vi "Init.vi"(0 "Session Handle in":T1, 11 "error in (no error)":errorcluster) -> (4 "Session Handle out":T1, 15 "error out":errorcluster)   [LabVIEW 2019, in "SmartScopeDriver.lvclass"]
doc: "Initializes the Smart Scope."
uses:
  SmartScopeDriver.lvclass
  Typedefs/Session Handle.ctl
  SmartScopeDriver.lvclass/SmartScopeDriver.ctl
  Scope Driver/LabNation Scope Driver.lvlib
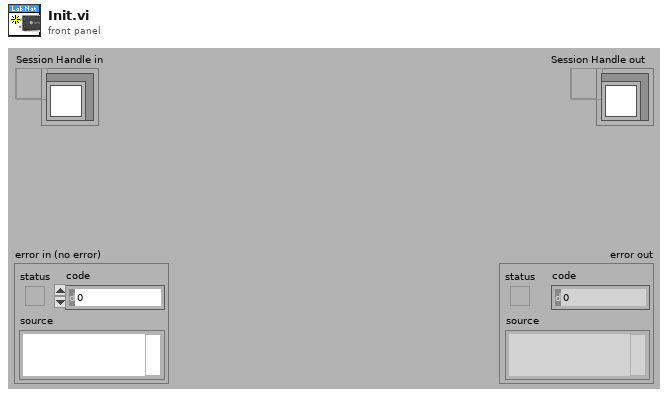
[diagram p1: front panel]
types:
  T1 = typedef "SmartScopeDriver.lvclass/Session Handle.ctl" = refnum<data-value>
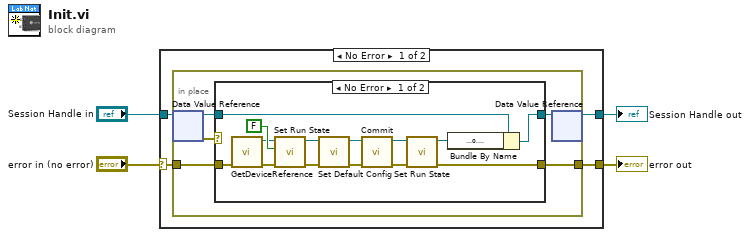
[diagram p0: block diagram]
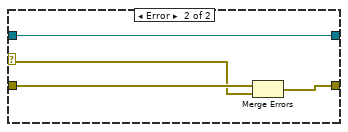
[diagram p2: hidden frame]
diagram:
  n1 = case shown="No Error" "error in (no error)" {
    selector: "error in (no error)" -> [w6 w32]
    tunnel: "Session Handle in" -> [w8 w33]
    tunnel: [w7 w33] -> w3
    tunnel: [w5 w32] -> w2
    frame No Error {
      n2 = in-place {
        in-place-border: w6 -> [w9]
        in-place-border: [w12] -> w5
        n3 = in-place-dvr #1(w8) -> (w13:refnum<class "SmartScopeDriver.lvclass">, w10:errorcluster)
        n4 = case shown="No Error" w10 {
          selector: w10 -> [_ w30]
          tunnel: w13 -> [w15 w28]
          tunnel: [w16 w29] -> w12
          tunnel: [w14 w28] -> w11
          tunnel: w9 -> [w27 w31]
          frame No Error {
            n5 = call "GetDeviceReference.vi"("error in (no error)"=w27) -> ("error out"=w24:errorcluster, "MainDevice Reference"=w25:refnum<k24>)  [unwired: 9 in]
            n6 = call "Set Run State.vi"("error in (no error)"=w24, "RunState(T)"=FALSE ("RunState"), "reference in"=w25) -> ("error out"=w22:errorcluster, "reference out"=w23:refnum<k24>)  [unwired: 7 in]
            n7 = call "Set Default Config.vi"("error in (no error)"=w22, "reference in"=w23) -> ("error out"=w20:errorcluster, "reference out"=w21:refnum<k24>)  [unwired: 8 in]
            n8 = call "Commit.vi"("error in (no error)"=w20, "reference in"=w21) -> ("error out"=w19:errorcluster, "reference out"=w18:refnum<k24>)  [unwired: 8 in]
            n9 = call "Set Run State.vi"("error in (no error)"=w19, "reference in"=w18) -> ("error out"=w16:errorcluster, "reference out"=w17:refnum<k24>)  [unwired: 8 in]
            n10 = Bundle By Name(cluster=w15, "reference"=w17) -> (w14:refnum<class "SmartScopeDriver.lvclass">)
          }
          frame Error {
            n11 = Merge Errors(w31, w30) -> (w29:errorcluster)
          }
        }
        n12 = in-place-dvr #1(w11) -> (w7:T1)  [unwired: 1 out]
      }
    }
    frame Error {
    }
  }
  "Session Handle out" <- w3
  "error out" <- w2
